vi "Player Info.vi"(11 "Hungry Wolf in":refnum<class "Hungry Wolf.lvclass">) -> (1 "Victory Speech":string, 2 "Name":string, 3 "Hungry Wolf out":refnum<class "Hungry Wolf.lvclass">)   [LabVIEW 2015, in "Hungry Wolf.lvclass"]
uses:
  Hungry Wolf.lvclass
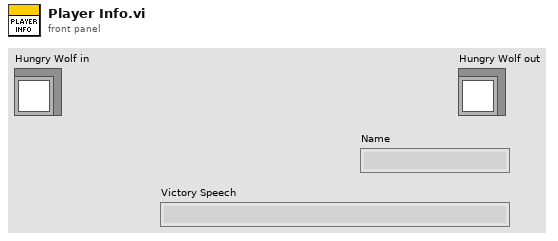
[diagram p1: front panel]
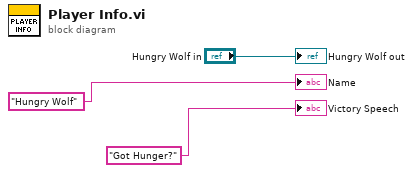
[diagram p0: block diagram]
diagram:
  "Hungry Wolf out" <- "Hungry Wolf in"
  "Name" <- "Hungry Wolf" ("Name")
  "Victory Speech" <- "Got Hunger?" ("Victory Speech")
